vi "HEWH_Power ON.vi"(8 "error in (no error)":errorcluster) -> (0 "error out":errorcluster, 3 "ON or OFF":bool)   [LabVIEW 2016]
panel:
  in  "Complete":bool
  in  "Power":string(combo)
  out "Description":string="HEWH Power Status"
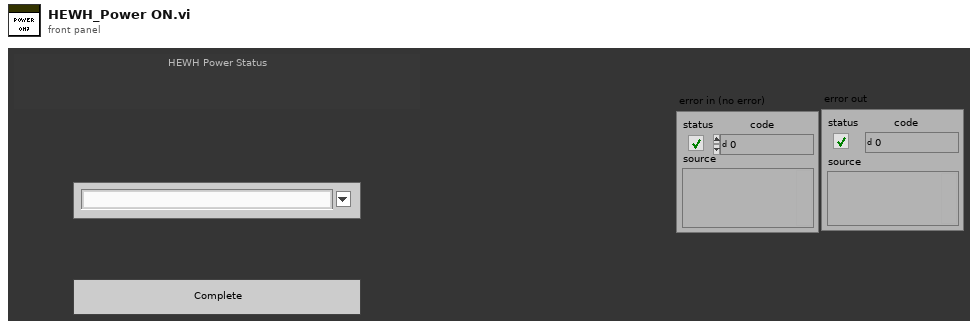
[diagram p1: front panel]
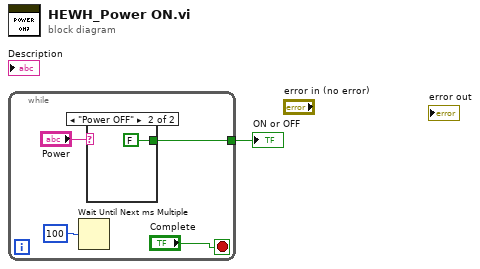
[diagram p0: block diagram]
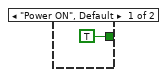
[diagram p2: hidden frame]
diagram:
  n1 = while {
    tunnel: [w4] -> w1
    stop <- "Complete" stop-if-true
    n2 = Wait Until Next ms Multiple(millisecond multiple=u32 100) -> ()  [unwired: 1 out]
    n3 = case shown="\"Power OFF\"" "Power" {
      tunnel: [TRUE FALSE] -> w4
      frame "Power ON", Default {
      }
      frame "Power OFF" {
      }
    }
  }
  "ON or OFF" <- w1
